vi "New SwipeScrollListbox.vi"(11 "Reference":refnum<vi>) -> (0 "error out":errorcluster, 3 "SwipeScrollListbox out":refnum<class "SwipeScrollListbox.lvclass">)   [LabVIEW 2020, in "SwipeScrollListbox.lvclass"]
doc: "The Constructor Method is the method that instantiates the new QControl Class. It is named \"New\" and then the name of the QControl Class (i.e. New StatusHistory.vi). Its only input is the control reference that the new QControl Class will control. \n\nThe Constructor will then:\n1. Cast the reference to \"Generic\" and call the Load Reference Method to load the control reference to the class private data \n2. Call the Load State Data Method which loads the State Data DVR to the class private data\n3. Call the Initialize Method to perform any initialization and start any other references used by the QControl Class and launch the Event Handler\n\nThe output of the Constructor Method is the QControl Class Wire. This wire should be handled and passed just like the reference of a basic control/indicator. <b>Any manipulation of the control after the Constructor Method should use Properties or Methods on this wire or handle UI Logic in the Event Handler.</b>\n<b> </b> <b> </b>\n©2016 Q Software Innovations, LLC (QSI)\nwritten by Quentin Alldredge\nproduced in LabVIEW 2015\n\nsupport@qsoftwareinnovations.com\nwww.qsoftwareinnovations.com\n\nAll rights reserved.\n\nRedistribution and use in source and binary forms, with or without modification, are permitted provided that the following conditions are met:\n\n * Redistributions of source code must retain the above copyright notice, this list of conditions and the following disclaimer.\n * Redistributions in binary form must reproduce the above copyright notice, this list of conditions and the following disclaimer in the documentation and/or other materials provided with the distribution.\n * Neither the name of Q Software Innovations, LLC. nor the names of its contributors may be used to endorse or promote products derived from this software without specific prior written permission.\n\nTHIS SOFTWARE IS PROVIDED BY THE COPYRIGHT HOLDERS AND CONTRIBUTORS \"AS IS\" AND ANY EXPRESS OR IMPLIED WARRANTIES, INCLUDING, BUT NOT LIMITED TO, THE IMPLIED WARRANTIES OF MERCHANTABILITY AND FITNESS FOR A PARTICULAR PURPOSE ARE DISCLAIMED. IN NO EVENT SHALL THE COPYRIGHT OWNER OR CONTRIBUTORS BE LIABLE FOR ANY DIRECT, INDIRECT, INCIDENTAL, SPECIAL, EXEMPLARY, OR CONSEQUENTIAL DAMAGES (INCLUDING, BUT NOT LIMITED TO, PROCUREMENT OF SUBSTITUTE GOODS OR SERVICES; LOSS OF USE, DATA, OR PROFITS; OR BUSINESS INTERRUPTION) HOWEVER CAUSED AND ON ANY THEORY OF LIABILITY, WHETHER IN CONTRACT, STRICT LIABILITY, OR TORT (INCLUDING NEGLIGENCE OR OTHERWISE) ARISING IN ANY WAY OUT OF THE USE OF THIS SOFTWARE, EVEN IF ADVISED OF THE POSSIBILITY OF SUCH DAMAGE."
uses:
  SwipeScrollListbox.lvclass
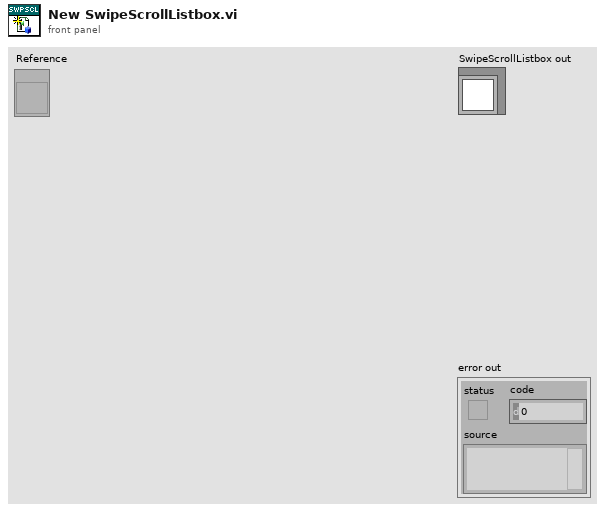
[diagram p1: front panel]
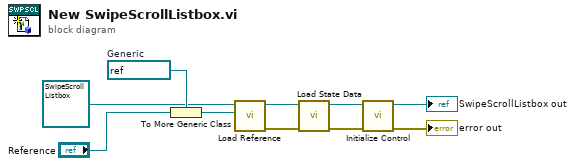
[diagram p0: block diagram]
diagram:
  w9 = refnum<vi> refnum  # Generic
  n1 = To More Generic Class(target class=w9, reference="Reference") -> (generic class reference=w10:refnum<vi>)
  n2 = call-dynamic "Load Reference.vi"("Reference"=w10, "SwipeScrollListbox in"=refnum<class "SwipeScrollListbox.lvclass"> refnum ("SwipeScrollListbox.lvclass")) -> ("error out"=w6:errorcluster, "SwipeScrollListbox out"=w3:refnum<class "SwipeScrollListbox.lvclass">)  [unwired: 8 in]
  n3 = call-dynamic "Load State Data.vi"("error in (no error)"=w6, "SwipeScrollListbox in"=w3) -> ("error out"=w4:errorcluster, "SwipeScrollListbox out"=w2:refnum<class "SwipeScrollListbox.lvclass">)  [unwired: 8 in]
  n4 = call-dynamic "Initialize Control.vi"("error in (no error)"=w4, "SwipeScrollListbox in"=w2) -> ("error out"=→"error out":errorcluster, "SwipeScrollListbox out"=→"SwipeScrollListbox out":refnum<class "SwipeScrollListbox.lvclass">)  [unwired: 8 in]
